vi "Stereo - Grid Coverage.vi"(8 "error in (no error)":errorcluster, 10 "Grid Images":T4(array[cluster]), 11 "Image in":T1) -> (0 "error out":errorcluster, 3 "Image out":T1)   [LabVIEW 2019]
doc: "Computes a grid coverage based on the Grid Images input array. The result is stored in the image provided as an input."
uses:
  <vilib>/vision/Image Controls.llb/IMAQ Image.ctl
  <vilib>/vision/Calibration.llb/Calibration Reference Points.ctl
  <vilib>/vision/NI_Vision_Development_Module.lvlib
  <vilib>/gmath/NI_Gmath.lvlib
panel:
  # "Overview: Computes a grid coverage based on the Grid Images input array.\n                     The result is stored in the image provided as an input."
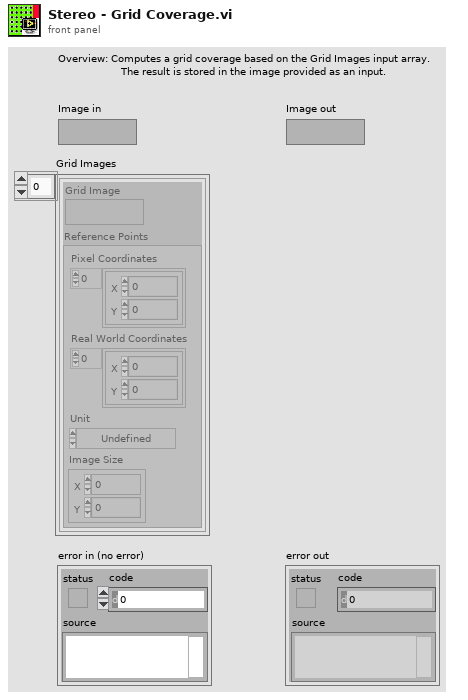
[diagram p1: front panel]
types:
  T1 = typedef "IMAQ Image.ctl" = refnum<image>
  T2 = typedef "Calibration Reference Points.ctl" = cluster{"Pixel Coordinates":cluster{"X":dbl, "Y":dbl}[], "Real World Coordinates":cluster{"X":dbl, "Y":dbl}[], "Unit":T3, "Image Size":cluster{"X":u32, "Y":u32}}
  T3 = typedef "Image Unit" = enum32{"Undefined", "Angström", "Micrometer", "Millimeter", "Centimeter", "Meter", "Kilometer", "Microinch", "Inch", "Feet", "Nautical miles", "Standard miles", "Steps"}
  T4 = cluster{"Grid Image":T1, "Reference Points":T2}[]
  T5 = enum16{"arithmetic", "geometric", "harmonic", "trimmed", "median"}
  T6 = cluster{cluster{"X":dbl, "Y":dbl}, cluster{"X":dbl, "Y":dbl}}
  T7 = cluster{cluster{"X":dbl, "Y":dbl}, cluster{"X":dbl, "Y":dbl}}[]
  T8 = cluster{"histogram":u32[], "Minimal Value":sgl, "Maximal Value":sgl, "Starting Value":sgl, "Interval Width":sgl, "Mean Value":sgl, "Standard  Variation":sgl, "Area (pixels)":i32}
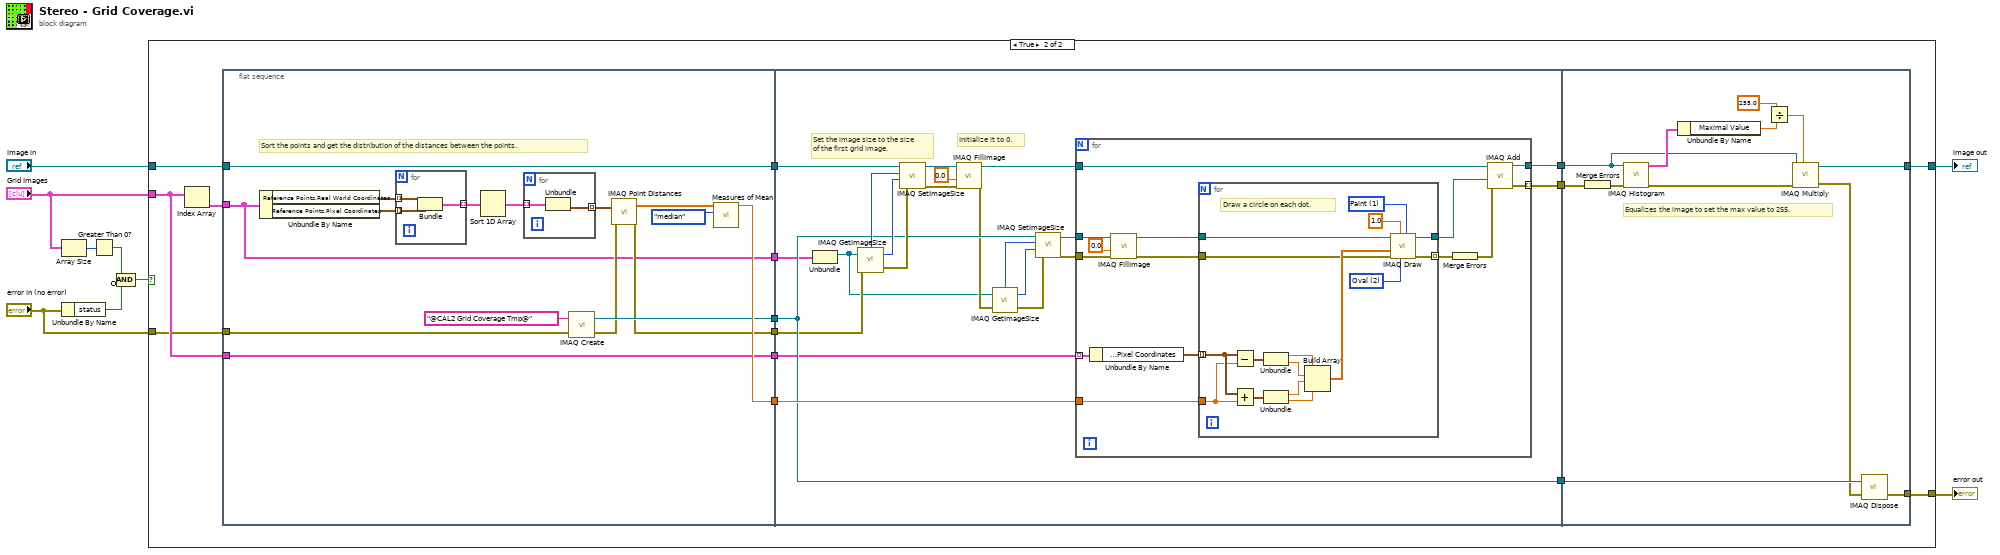
[diagram p0: block diagram]
diagram:
  n1 = Array Size(array="Grid Images") -> (size(s)=w5:i32)
  n2 = Unbundle By Name("error in (no error)") -> ("status"=w3:bool)
  n3 = Greater Than 0?(x=w5) -> (x > 0?=w4:bool)
  n4 = Compound Arithmetic op=AND(w4, invert w3) -> (w2:bool)
  n5 = case shown="True" w2 {
    tunnel: [w10 w26] -> w9
    tunnel: "Grid Images" -> [_ w24]
    tunnel: "Image in" -> [w11 w23]
    tunnel: [w11 w22] -> w7
    tunnel: "error in (no error)" -> [w10 w12]
    frame False {
    }
    frame True {
      n6 = Index Array(array=w24) -> (element=w25:cluster{"Grid Image":T1, "Reference Points":T2})  [unwired: 1 in]
      n7 = flat-sequence {
        tunnel: w24 -> [w30]
        tunnel: [w30] -> w21
        tunnel: w25 -> [w27]
        tunnel: [w27] -> w20
        tunnel: w23 -> [w29]
        tunnel: [w29] -> w19
        tunnel: [w37] -> w18
        tunnel: [w35] -> w17
        tunnel: [w34] -> w16
        tunnel: w12 -> [w28]
        tunnel: w21 -> [w50]
        tunnel: w20 -> [w52]
        tunnel: w19 -> [w49]
        tunnel: w18 -> [w59]
        tunnel: w17 -> [w58]
        tunnel: [w58] -> w15
        tunnel: [w57] -> w14
        tunnel: w16 -> [w56]
        tunnel: [w53] -> w13
        tunnel: [w100] -> w26
        tunnel: [w103] -> w22
        tunnel: w15 -> [w109]
        tunnel: w14 -> [w108]
        tunnel: w13 -> [w104]
        frame #0 {
          # "Sort the points and get the distribution of the distances between the points."
          n8 = Unbundle By Name(w27) -> ("Reference Points.Real World Coordinates"=w33:cluster{"X":dbl, "Y":dbl}[], "Reference Points.Pixel Coordinates"=w32:cluster{"X":dbl, "Y":dbl}[])
          n9 = for {
            tunnel: w32 -> [w45] mode=indexing
            tunnel: [w44] -> w39 mode=indexing
            tunnel: w33 -> [w43] mode=indexing
            n10 = Bundle(w43, w45) -> (w44:T6)  [unwired: 1 out]
          }
          n11 = Sort 1D Array(array=w39) -> (sorted array=w40:T7)
          n12 = for {
            tunnel: w40 -> [w47] mode=indexing
            tunnel: [w46] -> w41 mode=indexing
            n13 = Unbundle(w47) -> (w46:cluster{"X":dbl, "Y":dbl})  [unwired: 1 out]
          }
          n14 = call "IMAQ Create"("Image Name"="@CAL2 Grid Coverage Tmp@", "error in (no error)"=w28) -> ("New Image"=w35:T1, "error out"=w31:errorcluster)  [unwired: 2 in, 1 out]
          n15 = call "IMAQ Point Distances"("Points"=w41, "error in (no error)"=w31) -> ("Distances"=w42:sgl[], "error out"=w34:errorcluster)  [unwired: 3 out]
          n16 = call <vilib>:"Measures of Mean.vi"("type"=T5."median", "x array"=w42) -> ("mean value"=w37:dbl)  [unwired: 1 in, 8 out]
        }
        frame #1 {
          # "Initialize it to 0."
          # "Set the image size to the size of the first grid image."
          n17 = Unbundle(w52) -> ("Grid Image"=w51:T1)  [unwired: 1 out]
          n18 = call "IMAQ GetImageSize"("Image"=w51, "error in (no error)"=w56) -> ("Y Resolution"=w68:i32, "X Resolution"=w69:i32, "error out"=w67:errorcluster)  [unwired: 2 out]
          n19 = call "IMAQ SetImageSize"("error in (no error)"=w67, "Y Resolution"=w68, "X Resolution"=w69, "Image"=w49) -> ("error out"=w48:errorcluster, "Image Out"=w65:T1)  [unwired: 1 out]
          n20 = call "IMAQ FillImage"("error in (no error)"=w48, "Pixel Value (U8, U16, I16, Float)"=sgl 0.0, "Image"=w65) -> ("error out"=w55:errorcluster, "Image Out"=w66:T1)  [unwired: 4 in, 3 out]
          n21 = call "IMAQ GetImageSize"("Image"=w51, "error in (no error)"=w55) -> ("Y Resolution"=w62:i32, "X Resolution"=w63:i32, "error out"=w61:errorcluster)  [unwired: 2 out]
          n22 = call "IMAQ SetImageSize"("error in (no error)"=w61, "Y Resolution"=w62, "X Resolution"=w63, "Image"=w58) -> ("error out"=w54:errorcluster, "Image Out"=w60:T1)  [unwired: 1 out]
          n23 = for {
            tunnel: w66 -> [w81]
            tunnel: [w80] -> w57
            tunnel: w59 -> [w83]
            tunnel: w60 -> [w82]
            tunnel: w54 -> [w79]
            tunnel: [w78] -> w53 mode=indexing
            tunnel: w50 -> [w72] mode=indexing
            n24 = Unbundle By Name(w72) -> ("Reference Points.Pixel Coordinates"=w71:cluster{"X":dbl, "Y":dbl}[])
            n25 = call "IMAQ FillImage"("error in (no error)"=w79, "Pixel Value (U8, U16, I16, Float)"=sgl 0.0, "Image"=w82) -> ("error out"=w74:errorcluster, "Image Out"=w76:T1)  [unwired: 4 in, 3 out]
            n26 = for {
              tunnel: w71 -> [w95] mode=indexing
              tunnel: w76 -> [w99]
              tunnel: [w96] -> w75
              tunnel: w83 -> [w94]
              tunnel: w74 -> [w85]
              tunnel: [w84] -> w70 mode=indexing
              w97 = u16 2 items=["Line", "Rectangle", "Oval"] ("Shape to draw")
              w98 = u16 1 items=["Frame", "Paint", "Invert Frame", "Invert Paint"] ("Draw Mode")
              # "Draw a circle on each dot."
              n27 = Subtract(x=w95, y=w94) -> (x-y=w93:cluster{"X":dbl, "Y":dbl})
              n28 = Add(x=w95, y=w94) -> (x+y=w92:cluster{"X":dbl, "Y":dbl})
              n29 = Unbundle(w93) -> ("X"=w91:dbl, "Y"=w90:dbl)
              n30 = Unbundle(w92) -> ("X"=w89:dbl, "Y"=w88:dbl)
              n31 = Build Array(w91, w90, w89, w88) -> (w87:dbl[])
              n32 = call "IMAQ Draw"("Draw Mode"=w98, "Shape to draw"=w97, "Pixel Color"=sgl 1.0, "error in (no error)"=w85, "Coordinates"=w87, "Image Src"=w99) -> ("error out"=w84:errorcluster, "Image Dst Out"=w96:T1)  [unwired: 1 in, 3 out]
            }
            n33 = Merge Errors(w70) -> (w73:errorcluster)
            n34 = call "IMAQ Add"("Image Src A"=w81, "Image Src B"=w75, "error in (no error)"=w73) -> ("Image Dst Out"=w80:T1, "error out"=w78:errorcluster)  [unwired: 2 in, 2 out]
          }
        }
        frame #2 {
          # "Equalizes the image to set the max value to 255."
          n35 = Merge Errors(w104) -> (w110:errorcluster)
          n36 = call "IMAQ Histogram"("error in (no error)"=w110, "Image"=w108) -> ("error out"=w102:errorcluster, "Histogram Report"=w111:T8)  [unwired: 3 in, 5 out]
          n37 = Unbundle By Name(w111) -> ("Maximal Value"=w105:sgl)
          n38 = Divide(x=sgl 255.0 ("Constant"), y=w105) -> (x/y=w106:sgl)
          n39 = call "IMAQ Multiply"("Image Src A"=w108, "Constant"=w106, "error in (no error)"=w102) -> ("Image Dst Out"=w103:T1, "error out"=w101:errorcluster)  [unwired: 2 in, 2 out]
          n40 = call "IMAQ Dispose"("Image"=w109, "error in (no error)"=w101) -> ("error out"=w100:errorcluster)  [unwired: 1 in, 3 out]
        }
      }
    }
  }
  "error out" <- w9
  "Image out" <- w7
